vi "Read Brucker Instances.vi"(8 "error in (no error)":errorcluster, 11 "OSSP_Problem in":refnum<class "OSSP_Problem.lvclass">) -> (0 "error out":errorcluster, 3 "OSSP_Problem out":refnum<class "OSSP_Problem.lvclass">)   [LabVIEW 2013, in "OSSP_Problem.lvclass"]
uses:
  OSSP_Problem.lvclass
  OSSP_Problem.lvclass/OSSP_Problem.ctl
panel:
  out "Processing Times":u16[][](array[numeric])
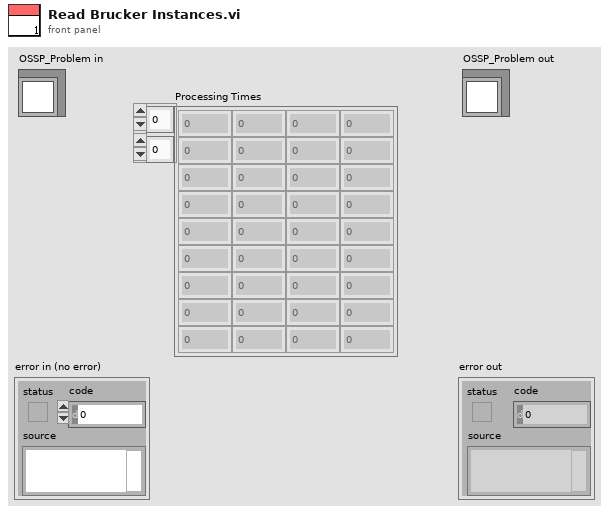
[diagram p1: front panel]
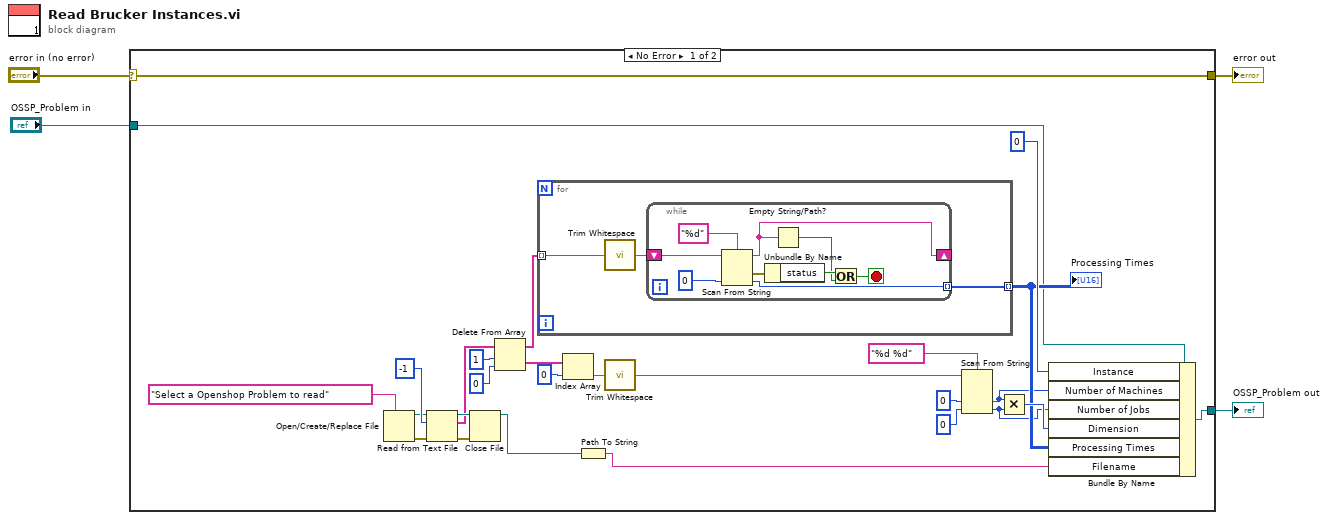
[diagram p0: block diagram]
diagram:
  n1 = case shown="No Error" "error in (no error)" {
    selector: "error in (no error)" -> [w31 w45]
    tunnel: [w31 w45] -> w3
    tunnel: [w17 w44] -> w1
    tunnel: "OSSP_Problem in" -> [w18 w44]
    frame No Error {
      n2 = Open/Create/Replace File(prompt="Select a Openshop Problem to read") -> (refnum out=w7:refnum<file>, error out=w26:errorcluster)  [unwired: 5 in, 1 out]
      n3 = Read from Text File(file (use dialog)=w7, count=-1, error in=w26) -> (refnum out=w28:refnum<file>, text=w25:string[], error out=w27:errorcluster)  [unwired: 1 in, 1 out]
      n4 = Close File(refnum=w28, error in=w27) -> (path=w6:path)  [unwired: 1 out]
      n5 = Delete From Array(array=w25, length=1, index=0) -> (deleted portion=w24:string[], array with subset deleted=w22:string[])
      n6 = for {
        tunnel: w22 -> [w33] mode=indexing
        tunnel: [w34] -> w19 mode=indexing
        n7 = call <vilib>:"Trim Whitespace.vi"("string"=w33) -> ("trimmed string"=w32:string)  [unwired: 1 in]
        n8 = while {
          shift-right: [w39] -> _
          shift-left: w32 -> [w43]
          tunnel: [w41] -> w34 mode=indexing
          stop <- w35 stop-if-true
          n9 = Scan From String(format string="%d", input string=w43, default 1=u16 0 ("default value 1")) -> (remaining string=w39:string, error out=w38:errorcluster, output 1=w41:u16)  [unwired: 2 in, 1 out]
          n10 = Unbundle By Name(w38) -> ("status"=w37:bool)
          n11 = Empty String/Path?(string/path=w39) -> (empty?=w36:bool)
          n12 = Or(x=w37, y=w36) -> (x .or. y?=w35:bool)
        }
      }
      "Processing Times" <- w19
      n13 = Index Array(array=w24, index=0) -> (element=w8:string)
      n14 = Path To String(path=w6) -> (string=w5:string)
      n15 = call <vilib>:"Trim Whitespace.vi"("string"=w8) -> ("trimmed string"=w16:string)  [unwired: 1 in]
      n16 = Scan From String(format string="%d %d", input string=w16, default 1=u8 0 ("default value 1"), default 2=u8 0 ("default value 2")) -> (output 1=w12:u8, output 2=w11:u8)  [unwired: 2 in, 3 out]
      n17 = Multiply(x=w12, y=w11) -> (x*y=w20:u8)
      n18 = Bundle By Name(cluster=w18, "Instance"=u8 0, "Number of Machines"=w12, "Number of Jobs"=w11, "Dimension"=w20, "Processing Times"=w19, "Filename"=w5) -> (w17:refnum<class "OSSP_Problem.lvclass">)
    }
    frame Error {
    }
  }
  "error out" <- w3
  "OSSP_Problem out" <- w1
